vi "Engine-In.vi"(8 "error in (no error)":errorcluster, 11 "DSI Reference":refnum<class "DCM-DSI.lvclass">) -> (0 "error out":errorcluster, 3 "DSI Reference":refnum<class "DCM-DSI.lvclass">)   [LabVIEW 2016, in "DSI-RT.lvlib"]
uses:
  DSI-RT.lvlib
  Classes/DCM-DSI/DCM-DSI.lvclass
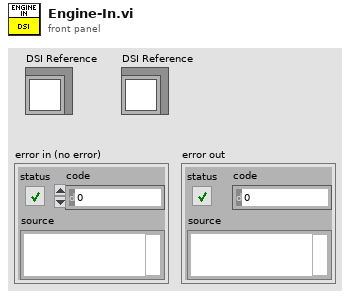
[diagram p1: front panel]
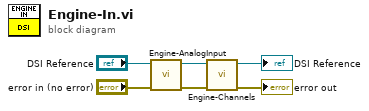
[diagram p0: block diagram]
diagram:
  n1 = call "Engine-AnalogInput.vi"("error in (no error)"="error in (no error)", "DSI Reference"="DSI Reference") -> ("error out"=w2:errorcluster, "DSI Reference"=w5:refnum<class "DCM-DSI.lvclass">)  [unwired: 8 in]
  n2 = call "Engine-Channels.vi"("error in (no error)"=w2, "DSI Reference"=w5) -> ("error out"=→"error out":errorcluster, "DSI Reference"=→"DSI Reference":refnum<class "DCM-DSI.lvclass">)  [unwired: 8 in]
